vi "整型数正则表达式（精确整型数，单词）.vi"(8 "error in (no error)":errorcluster caption="错误输入（无错误）", 11 "整型数":i32) -> (0 "error out":errorcluster caption="错误输出", 3 "正则表达式":string)   [LabVIEW 2011]
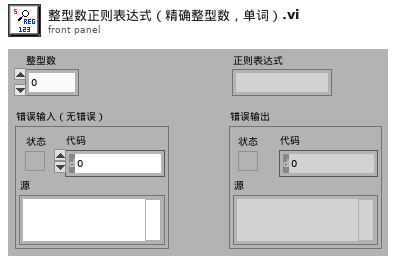
[diagram p1: front panel]
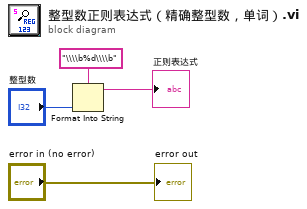
[diagram p0: block diagram]
diagram:
  n1 = Format Into String(format string="\\\\b%d\\\\b" ("格式字符串"), "整型数") -> (resulting string=→"正则表达式":string)  [unwired: 2 in, 1 out]
  "error out" <- "error in (no error)"
